vi "Wait for Stage.vi"(8 "error in (no error)":errorcluster, 11 "Recipe Process in":refnum<class "Recipe Process.lvclass">) -> (0 "error out":errorcluster, 3 "Recipe Process out":refnum<class "Recipe Process.lvclass">)   [LabVIEW 2022 SP3, in "Recipe Process.lvlib" / "Recipe Process.lvclass"]
uses:
  Recipe Process.lvclass
  Recipe Process.lvclass/Recipe Process.ctl
  XY Stage/Process Actor/Process Framework/Process State Data/Process State Data.lvclass/Process State Data.ctl
  XY Stage/Process Actor/Process Framework/Process State Data/Accessor/Read Abort.vi
  XY Stage/Interfaces/2-Axis Stage API/2-Axis Stage Async API.lvclass
  XY Stage/Process Actor/Process Framework/Process State Data/Process State Data.lvclass
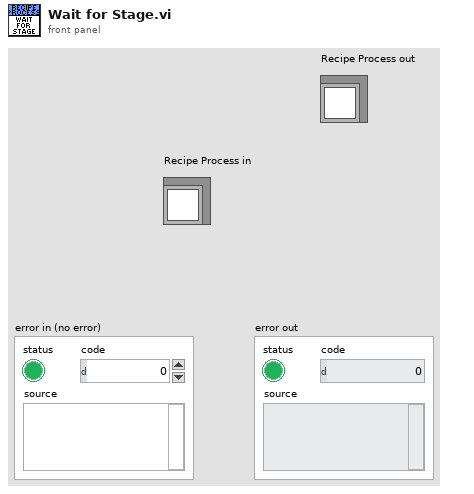
[diagram p1: front panel]
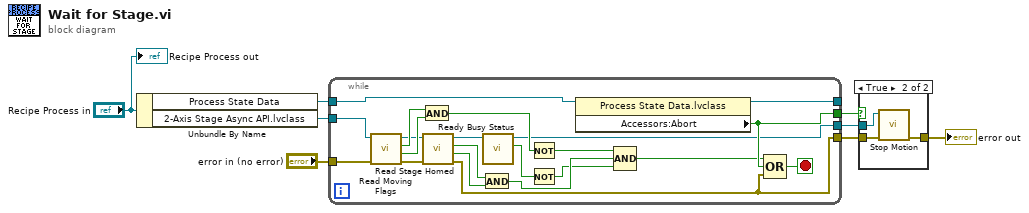
[diagram p0: block diagram]
diagram:
  n1 = Unbundle By Name("Recipe Process in") -> ("Process State Data"=w1:refnum<data-value>, "2-Axis Stage Async API.lvclass"=w2:refnum<class "2-Axis Stage Async API.lvclass">)
  n2 = while {
    tunnel: w2 -> [w29]
    tunnel: "error in (no error)" -> [w26]
    tunnel: w1 -> [w20]
    tunnel: [w9] -> w7
    tunnel: [w18] -> _
    tunnel: [w17] -> w5
    tunnel: [w10] -> w6
    stop <- w19 stop-if-true
    n3 = call-dynamic "Read Moving Flags.vi"("error in (no error)"=w26, "2-Axis Stage Status in"=w29) -> ("error out"=w23:errorcluster, "Y-Axis Moving"=w27:bool, "X-Axis Moving"=w28:bool, "2-Axis Stage Status out"=w24:refnum<class "2-Axis Stage Async API.lvclass">)  [unwired: 6 in]
    n4 = And(x=w28, y=w27) -> (x .and. y?=w25:bool)
    n5 = call-dynamic "Read Stage Homed.vi"("error in (no error)"=w23, "2-Axis Stage Status in"=w24) -> ("error out"=w9:errorcluster, "Y-Axis Homed"=w21:bool, "X-Axis Homed"=w22:bool, "2-Axis Stage Status out"=w13:refnum<class "2-Axis Stage Async API.lvclass">)  [unwired: 6 in]
    n6 = And(x=w22, y=w21) -> (x .and. y?=w15:bool)
    n7 = call-dynamic "Ready Busy Status.vi"("2-Axis Stage Status in"=w13) -> ("Busy"=w12:bool, "2-Axis Stage Status out"=w10:refnum<class "2-Axis Stage Async API.lvclass">)  [unwired: 8 in, 1 out]
    n8 = Not(x=w25) -> (.not. x?=w16:bool)
    n9 = Not(x=w12) -> (.not. x?=w11:bool)
    n10 = property class="Process State Data.lvclass"(reference=w20) -> (reference out=w18:refnum<data-value>, "Accessors:Abort"=w17:bool)  [unwired: 1 in, 1 out]
    n11 = Compound Arithmetic op=AND(w16, w15, w11) -> (w14:bool)
    n12 = Compound Arithmetic op=OR(w14, w17, w9) -> (w19:bool)
  }
  n13 = case shown="True" w5 {
    tunnel: w6 -> [_ w33]
    tunnel: w7 -> [w30 w32]
    tunnel: [w30 w31] -> w8
    frame False {
    }
    frame True {
      n14 = call-dynamic "Stop Motion.vi"("error in (no error)"=w32, "2-Axis Stage in"=w33) -> ("error out"=w31:errorcluster)  [unwired: 8 in, 1 out]
    }
  }
  "error out" <- w8
  "Recipe Process out" <- "Recipe Process in"
